vi "test_conv4.vi"() -> ()   [LabVIEW 2018]
uses:
  <vilib>/addons/Modulation/Digital/Channel Coding/MT Convolutional Encoder (Rate).vi
  <vilib>/addons/Modulation/Analog/support/mod_Set Error Source.vi
  <vilib>/addons/Modulation/Digital/Support/Common/Validators/mod_Validate Bit Stream.vi
  <vilib>/addons/Modulation/Digital/Channel Coding/Convolutional codes/mod_Convolutional encoder.vi
  <vilib>/addons/Modulation/Digital/Support/Common/Validators/mod_AWGN Validate.vi
  <vilib>/addons/Modulation/Digital/Impairments/subVIs/mod_createSeeds.vi
  <vilib>/addons/Modulation/Digital/Channel Coding/Convolutional codes/subVIs/mod_Generate encoder tap connections.vi
  <vilib>/addons/Modulation/Digital/Channel Coding/Convolutional codes/subVIs/mod_Perform convolutional encoding.vi
  <vilib>/addons/Modulation/Digital/Channel Coding/Block codes/subVIs/mod_Buffer block code info (I8).vi
  <vilib>/addons/Modulation/Digital/Channel Coding/Convolutional codes/subVIs/mod_Generate valid reset (convolutional, I8).vi
  <vilib>/addons/Modulation/Digital/Support/Common/Validators/mod_Validate Samples Per Symbol.vi
  <vilib>/addons/Modulation/Analog/support/Validators/mod_Validate Complex Waveform.vi
  <vilib>/addons/Modulation/Analog/support/Validators/mod_WFErrorHandler.vi
  <vilib>/addons/Modulation/Digital/Channel Coding/Convolutional codes/subVIs/mod_Select known generator matrix.vi
  <vilib>/addons/Modulation/Digital/Support/Common/Validators/mod_Validate Convolutional Encoder prms.vi
  <vilib>/addons/Modulation/Digital/Support/Common/Validators/mod_Generate Filter Coefficients Validate.vi
  <vilib>/addons/Modulation/Digital/General/subVIs/mod_Generate Filter Coefficients.vi
  <vilib>/addons/Modulation/Digital/General/MT Generate PSK System Parameters(M).vi
  <vilib>/addons/Modulation/Digital/General/subVIs/mod_Generate Bits PN Sequence.vi
  <vilib>/Analysis/1siggen.llb/Gaussian White Noise (obs 90).vi
  <vilib>/addons/Modulation/Digital/General/MT Apply Matched Filter (Generic).vi
  <vilib>/addons/Modulation/Digital/General/MT Map PSK Symbols to Bits.vi
  <vilib>/addons/Modulation/Digital/Channel Coding/MT Convolutional Decoder (Viterbi Hard Decision, Rate).vi
  <vilib>/addons/Modulation/niDMT.lvlib
panel:
  out "message":i8[](array[numeric])
  out "IQ Constellation":T1(graph)
  out "Dec":i8[](array[numeric])
  out "CAN":i8[](array[numeric])
  in  "Eb/N0 (10 dB)":dbl=10.0 format="%.2f"
  in  "Traceback Depth (D)":i32=20
  in  "Constraint Length (K)":i32=3
  in  "Rate (k/n)":enum16{"1/2", "1/3", "1/4", "2/3", "3/4"}(ring)
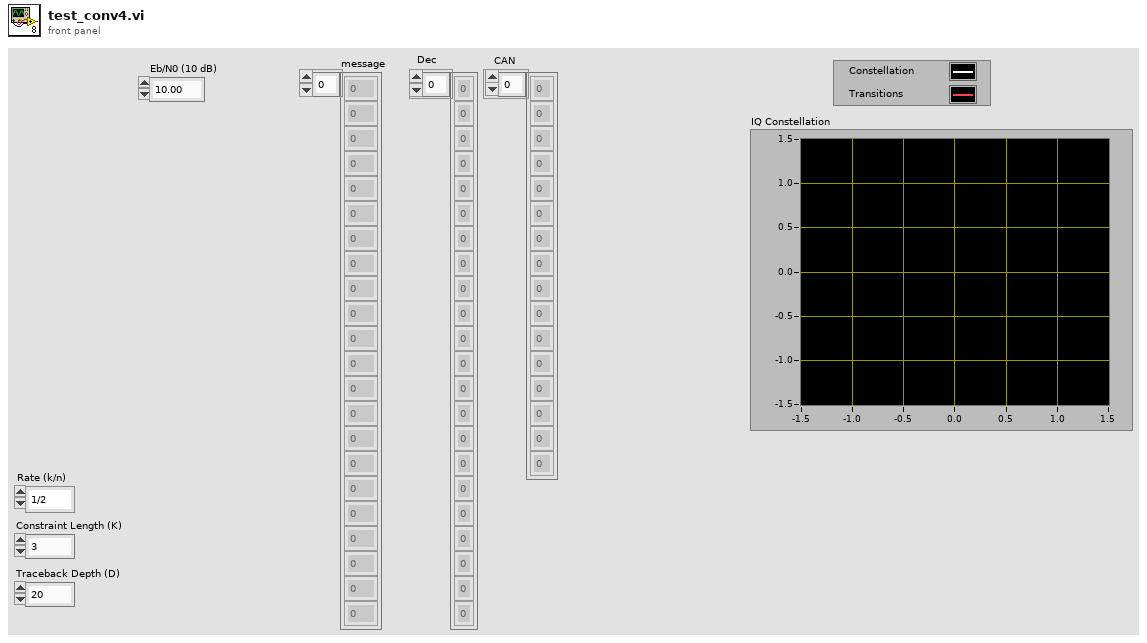
[diagram p1: front panel]
types:
  T1 = cluster{"Decimated Array":dbl[], "Decimated Array":dbl[]}[]
  T2 = enum16{"none", "Raised Cosine", "Root Raised Cos", "Gaussian"}
  T3 = cluster{"samples per symbol (16)":i32, "symbol map":cdb[], "differential PSK":enum16{"disable", "enable"}, "PSK type":u16}
  T4 = typedef "niAMT.lvlib/Complex Data Waveform.ctl" = cluster{"t0":dbl, "dt":dbl, "Y":cdb[]}
  T5 = cluster{"constellation":dbl[], "oversampled data":dbl[]}[]
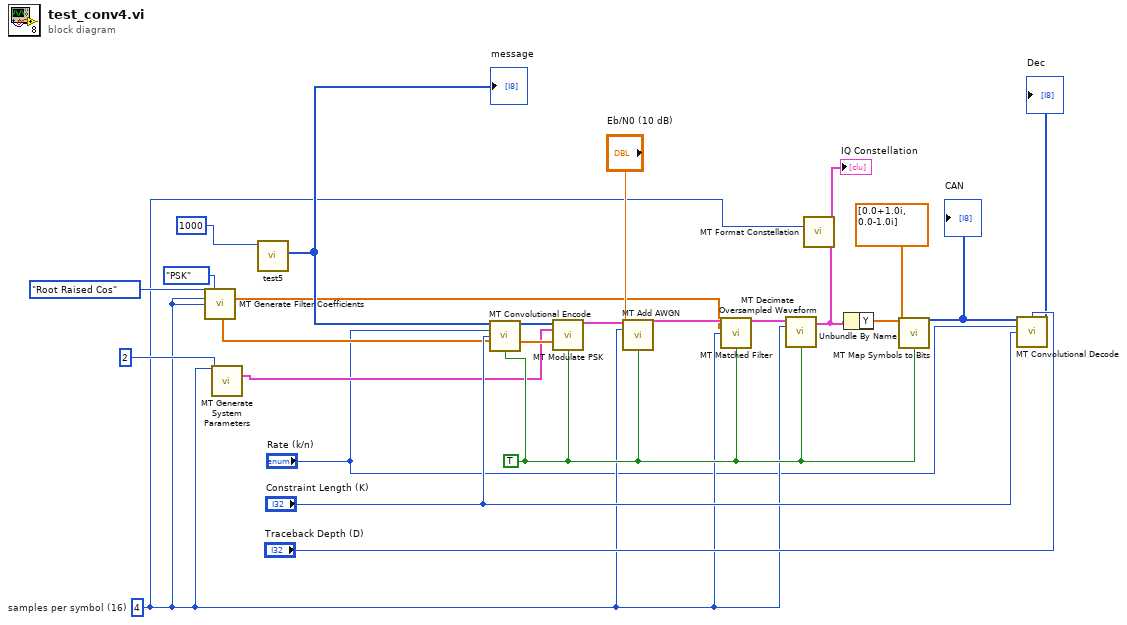
[diagram p0: block diagram]
diagram:
  w4 = 4  # samples per symbol (16)
  w15 = TRUE ("reset? (T)")
  n1 = call <vilib>:"MT Generate Filter Coefficients.vi"("pulse shaping filter (none)"=T2."Root Raised Cos", "modulation type"=enum16{"FSK", "PSK", "QAM", "MSK", "PAM", "ASK"}."PSK", "pulse shaping samples per symbol (16)"=w4, "matched samples per symbol (16)"=w4) -> ("pulse shaping filter coefficients"=w6:dbl[], "matched filter coefficients"=w5:dbl[])  [unwired: 9 in, 1 out]
  n2 = call-poly <vilib>:"MT Generate System Parameters.vi"("samples per symbol (16)"=w4, "M-PSK (4)"=2) -> ("PSK system parameters"=w3:T3)  [unwired: 11 in, 2 out]
  n3 = call "test5.vi"("k"=1000) -> ("output bit stream"=w17:i8[])  [unwired: 9 in, 1 out]
  "message" <- w17
  n4 = call-poly <vilib>:"MT Convolutional Encode.vi"("input bit stream"=w17, "rate (k/n)"="Rate (k/n)", "constraint length (K)"="Constraint Length (K)", "reset? (T)"=w15) -> ("output bit stream"=w23:i8[])  [unwired: 9 in, 2 out]
  n5 = call <vilib>:"MT Modulate PSK.vi"("input bit stream"=w23, "PSK system parameters"=w3, "pulse shaping filter coefficients"=w6, "reset? (T)"=w15) -> ("output complex waveform"=w24:T4)  [unwired: 9 in, 2 out]
  n6 = call <vilib>:"MT Add AWGN.vi"("input complex waveform"=w24, "samples per symbol (16)"=w4, "Eb/N0 (10 dB)"="Eb/N0 (10 dB)", "reset? (T)"=w15) -> ("output complex waveform"=w22:T4)  [unwired: 9 in, 2 out]
  n7 = call-poly <vilib>:"MT Matched Filter.vi"("input complex waveform"=w22, "matched filter coefficients"=w5, "samples per symbol (16)"=w4, "reset? (T)"=w15) -> ("output complex waveform"=w21:T4)  [unwired: 10 in, 1 out]
  n8 = call <vilib>:"MT Decimate Oversampled Waveform.vi"("input complex waveform"=w21, "decimation factor"=w4, "reset? (T)"=w15) -> ("output complex waveform"=w19:T4)  [unwired: 11 in, 1 out]
  n9 = call <vilib>:"MT Format Constellation.vi"("waveform"=w19, "samples per symbol"=w4) -> ("constellation graph"=→"IQ Constellation":T5)  [unwired: 12 in, 1 out]
  n10 = Unbundle By Name(w19) -> ("Y"=w20:cdb[])
  n11 = call-poly <vilib>:"MT Map Symbols to Bits.vi"("symbols"=w20, "symbol map"=cdb[] [0.0+1.0i, 0.0-1.0i], "reset? (T)"=w15) -> ("output bit stream"=w13:i8[])  [unwired: 11 in, 1 out]
  "CAN" <- w13
  n12 = call-poly <vilib>:"MT Convolutional Decode.vi"("input bit stream"=w13, "traceback depth (D)"="Traceback Depth (D)", "rate (k/n)"="Rate (k/n)", "constraint length (K)"="Constraint Length (K)") -> ("output bit stream"=→"Dec":i8[])  [unwired: 9 in, 2 out]
